vi "Get HW Config File Path.vi"(2 "Reset/Set File Path (F)?":bool, 7 "File Path":path=path "No Path Selected", 11 "Error":errorcluster) -> (8 "File Path":path, 15 "Error":errorcluster)   [LabVIEW 2025]
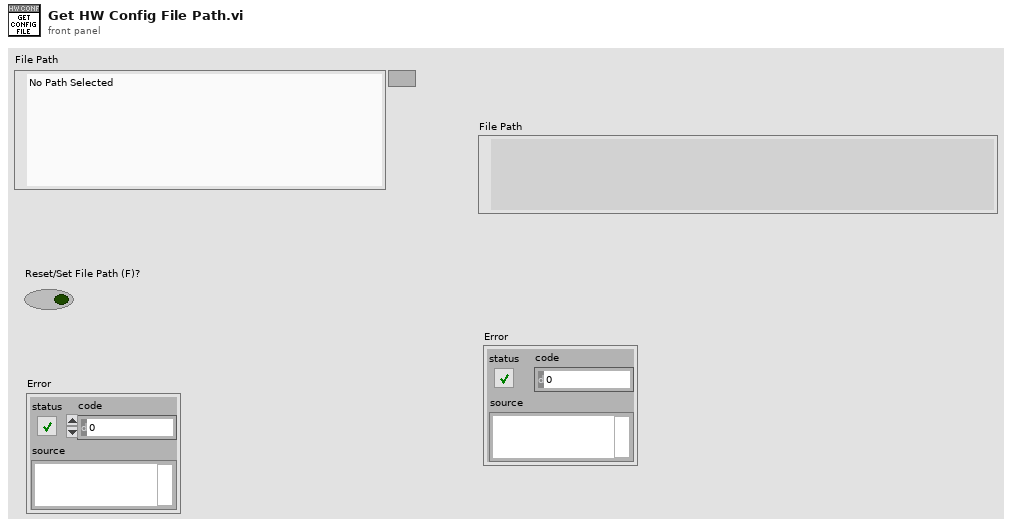
[diagram p1: front panel]
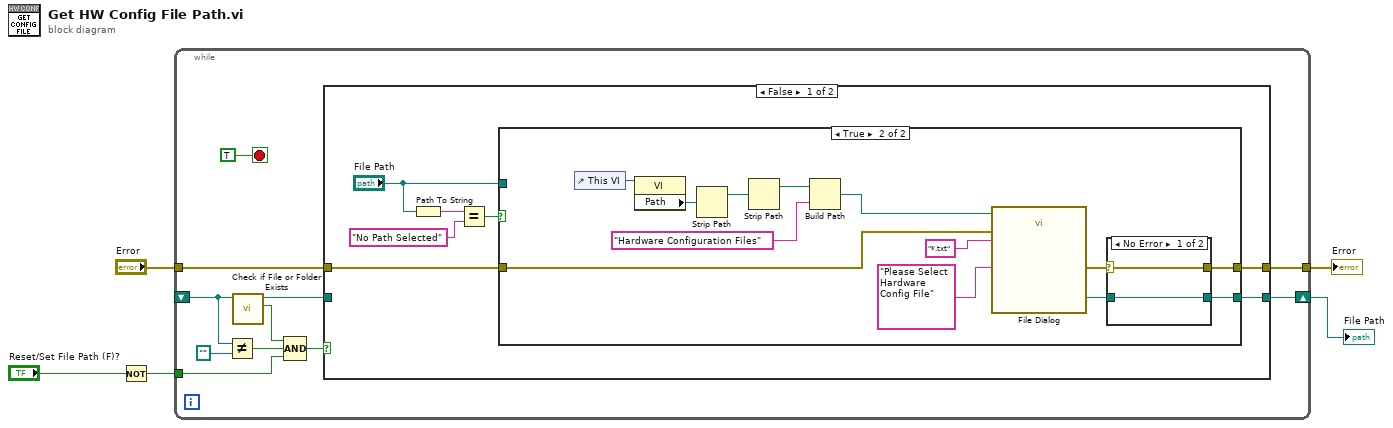
[diagram p0: block diagram]
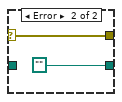
[diagram p3: hidden frame]
diagram:
  n1 = Not(x="Reset/Set File Path (F)?") -> (.not. x?=w2:bool)
  n2 = while {
    shift-right: [w15] -> w5
    shift-left: _ -> [w14]
    tunnel: [w11] -> w4
    tunnel: w2 -> [w8]
    tunnel: "Error" -> [w6]
    stop <- TRUE stop-if-true
    n3 = Not Equal?(x=w14, y=path "") -> (x != y?=w9:bool)
    n4 = call <vilib>:"Check if File or Folder Exists.vi"("path"=w14) -> ("file or folder exists?"=w10:bool, "dup path"=w12:path)  [unwired: 8 in, 1 out]
    n5 = Compound Arithmetic op=AND(w10, w9, w8) -> (w7:bool)
    n6 = case shown="False" w7 {
      tunnel: [w23 w44] -> w15
      tunnel: w12 -> [_ w44]
      tunnel: [w22 w43] -> w11
      tunnel: w6 -> [w17 w43]
      frame False {
        n7 = Path To String(path="File Path") -> (string=w21:string)
        n8 = Equal?(x=w21, y="No Path Selected") -> (x = y?=w19:bool)
        n9 = case shown="True" w19 {
          tunnel: [w25 w34] -> w23
          tunnel: [w24 w33] -> w22
          tunnel: "File Path" -> [w25 _]
          tunnel: w17 -> [w24 w32]
          frame False {
          }
          frame True {
            n10 = control-ref of="This VI"() -> (w28:refnum<vi>)
            n11 = property class="VI"(reference=w28) -> ("Path"=w29:path)  [unwired: 1 in, 2 out]
            n12 = Strip Path(path=w29) -> (stripped path=w27:path)  [unwired: 1 out]
            n13 = Strip Path(path=w27) -> (stripped path=w30:path)  [unwired: 1 out]
            n14 = Build Path(base path=w30, name or relative path="Hardware Configuration Files") -> (appended path=w26:path)
            n15 = call "File Dialog"("start path"=w26, "prompt"="Please Select Hardware Config File", "error in"=w32, "pattern (all files)"="*.txt") -> ("selected path"=w35:path, "error out"=w36:errorcluster)  [unwired: 8 in, 2 out]
            n16 = case shown="No Error" w36 {
              selector: w36 -> [w39 w41]
              tunnel: w35 -> [w40 _]
              tunnel: [w40 path ""] -> w34
              tunnel: [w39 w41] -> w33
              frame No Error {
              }
              frame Error {
              }
            }
          }
        }
      }
      frame True {
      }
    }
  }
  "File Path" <- w5
  "Error" <- w4
